vi "Slide through AVI frames.vi"(0 "AVI file path":path) -> (1 "Image":T1(plugin-control), 2 "Frame number":u32, 3 "Time index\n(hr : min : sec : ms)":string="0 : 0 : 0 : 0", 4 "Error out":errorcluster)   [LabVIEW 2015]
panel:
  out "N frames":u32
  out "frames per sec":u32
  in  "Stop":bool
  in  "Frame number control":u32(slide) max=134 step=1 scale=-1.0..134.0
  # "PN 23/12/2014"
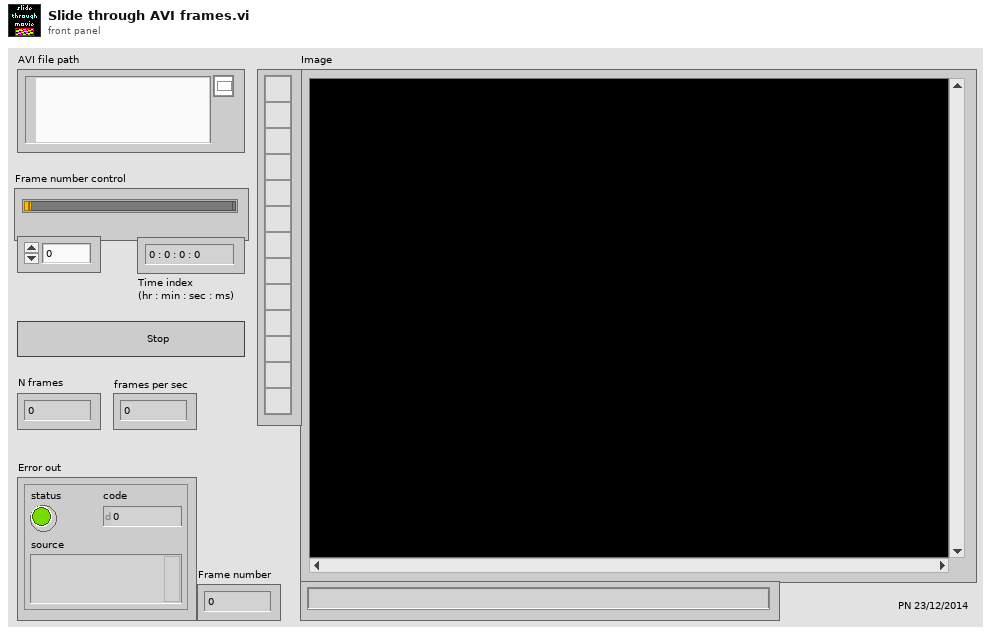
[diagram p1: front panel]
types:
  T1 = typedef "IMAQ Image.ctl" = refnum<image>
  T2 = typedef "IMAQ AVI2 Refnum.ctl" = refnum<k20>
  T3 = typedef "Image Type" = u32
  T4 = cluster{"Width":u32, "Height":u32, "Frames Per Second":u32, "Codec":string, "Has Data":bool}
  T5 = typedef "LVDateTimeRec.ctl" = cluster{"fractional second":dbl, "second":i32, "minute":i32, "hour":i32, "day of month":i32, "month":i32, "year":i32, "day of week":i32, "day of year":i32, "DST":i32}
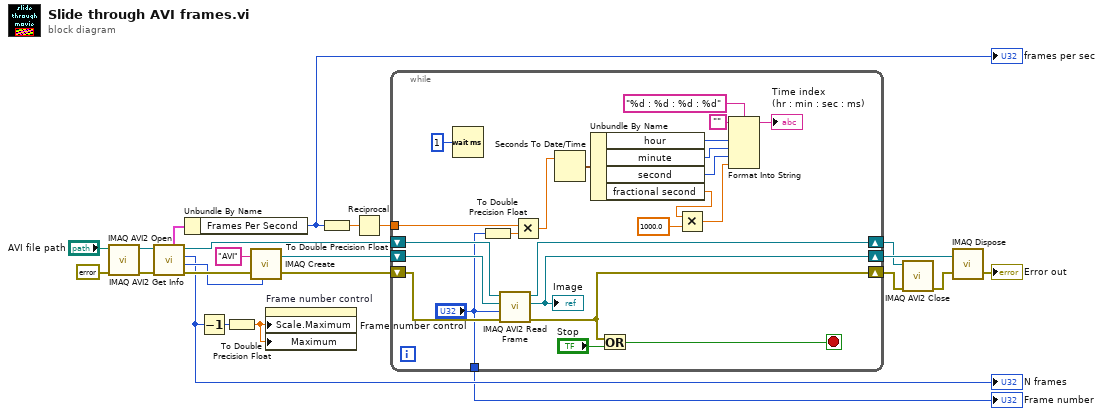
[diagram p0: block diagram]
diagram:
  n1 = call "IMAQ AVI2 Open"("error in (no error)"=errorcluster {"status"=FALSE, "code"=0, "source"=""}, "AVI File Path"="AVI file path") -> ("error out"=w19:errorcluster, "AVI Refnum"=w20:T2)  [unwired: 8 in]
  n2 = call "IMAQ AVI2 Get Info"("error in (no error)"=w19, "AVI Refnum"=w20) -> ("error out"=w18:errorcluster, "Image Type"=w17:T3, "Number of Frames"=w13:u32, "AVI Refnum (duplicate)"=w9:T2, "Frame Data"=w16:T4)  [unwired: 5 in]
  "N frames" <- w13
  n3 = Unbundle By Name(w16) -> ("Frames Per Second"=w15:u32)
  "frames per sec" <- w15
  n4 = Decrement(x=w13) -> (x-1=w3:u32)
  n5 = To Double Precision Float(number=w3) -> (double precision float=w1:dbl)
  n6 = call "IMAQ Create"("Image Name"="AVI", "Image Type"=w17, "error in (no error)"=w18) -> ("New Image"=w10:T1, "error out"=w11:errorcluster)  [unwired: 2 in]
  n7 = property on="Frame number control" class="Slide (strict)"("Scale.Maximum"=w1, "Maximum"=w1) -> ()  [unwired: 2 in, 2 out]
  n8 = To Double Precision Float(number=w15) -> (double precision float=w14:dbl)
  n9 = Reciprocal(x=w14) -> (1/x=w12:dbl)
  n10 = while {
    tunnel: w12 -> [w27]
    shift-right: [w43] -> w7
    shift-left: w11 -> [w44]
    shift-right: [w40] -> w8
    shift-left: w10 -> [w45]
    shift-right: [w39] -> w6
    shift-left: w9 -> [w46]
    tunnel: ["Frame number control"] -> w2
    stop <- w41 stop-if-true
    n11 = Wait (ms)(milliseconds to wait=u32 1) -> ()  [unwired: 1 out]
    n12 = To Double Precision Float(number="Frame number control") -> (double precision float=w26:dbl)
    n13 = call "IMAQ AVI2 Read Frame"("error in (no error)"=w44, "Frame Number"="Frame number control", "Image"=w45, "AVI Refnum"=w46) -> ("error out"=w43:errorcluster, "Image Out"=w40:T1, "AVI Refnum (duplicate)"=w39:T2)  [unwired: 5 in]
    "Image" <- w40
    n14 = Multiply(x=w27, y=w26) -> (x*y=w30:dbl)
    n15 = Seconds To Date/Time(time stamp (now)=w30) -> (date time rec=w31:T5)  [unwired: 1 in]
    n16 = Unbundle By Name(w31) -> ("hour"=w32:i32, "minute"=w33:i32, "second"=w34:i32, "fractional second"=w29:dbl)
    n17 = Or(x=w43, y="Stop") -> (x .or. y?=w41:bool)
    n18 = Multiply(x=w29, y=1000.0) -> (x*y=w28:dbl)
    n19 = Format Into String(format string="%d : %d : %d : %d", initial string="", w32, w33, w34, w28) -> (resulting string=→"Time index\n(hr : min : sec : ms)":string)  [unwired: 1 in, 1 out]
  }
  "Frame number" <- w2
  n20 = call "IMAQ AVI2 Close"("error in (no error)"=w7, "AVI Refnum"=w6) -> ("error out"=w5:errorcluster)  [unwired: 9 in]
  n21 = call "IMAQ Dispose"("Image"=w8, "error in (no error)"=w5) -> ("error out"=→"Error out":errorcluster)  [unwired: 4 in]
